vi "对称性.vi"(9 "索引":i32, 10 "定点":dbl, 11 "XY图":cluster{dbl[], dbl[]}[](graph)) -> (3 "对称性":dbl)   [LabVIEW 2020]
uses:
  <vilib>/Analysis/NI_AAL_Geometry.lvlib
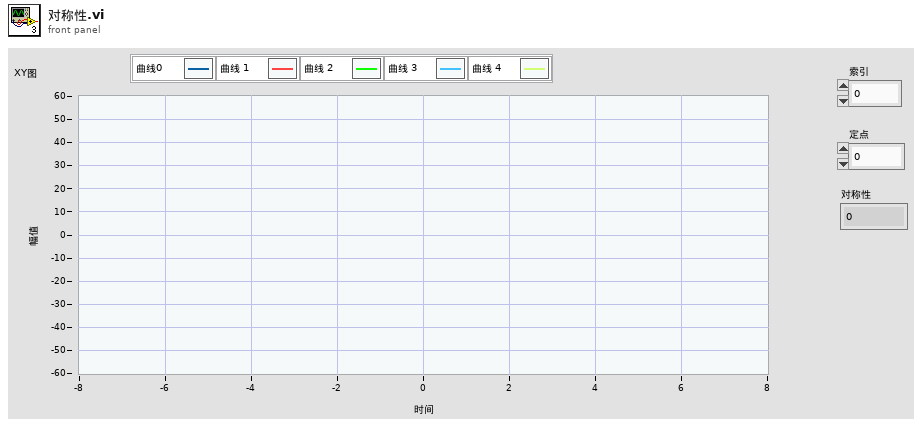
[diagram p1: front panel]
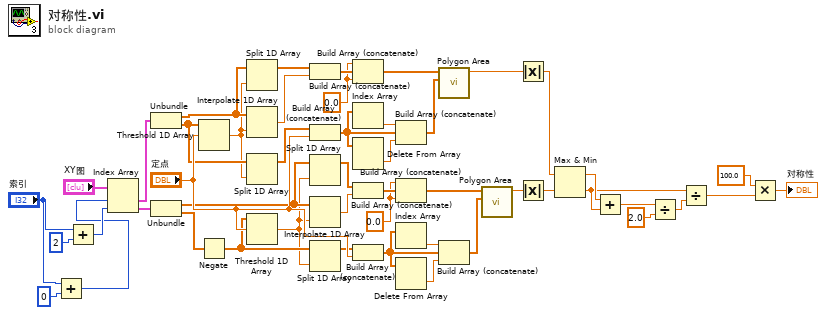
[diagram p0: block diagram]
diagram:
  w31 = 0.0
  w30 = 0.0
  n1 = Add(x="索引", y=0) -> (x+y=w2:i32)
  n2 = Add(x="索引", y=2) -> (x+y=w19:i32)
  n3 = Index Array(array="XY图", index #1=w2, index #2=w19) -> (element #1=w35:cluster{dbl[], dbl[]}, element #2=w21:cluster{dbl[], dbl[]})
  n4 = Unbundle(w35) -> (w32:dbl[], w34:dbl[])
  n5 = Unbundle(w21) -> (w13:dbl[], w33:dbl[])
  n6 = Threshold 1D Array(2:"定点", 3:w34) -> (0:w7:dbl)  [unwired: 1 in]
  n7 = Negate(x=w33) -> (-x=w12:dbl[])
  n8 = Split 1D Array(array=w32, index=w7) -> (first subarray=w11:dbl[])  [unwired: 1 out]
  n9 = Interpolate 1D Array(1:w7, 2:w32) -> (0:w6:dbl)
  n10 = Split 1D Array(array=w34, index=w7) -> (first subarray=w10:dbl[])  [unwired: 1 out]
  n11 = Threshold 1D Array(2:"定点", 3:w12) -> (0:w5:dbl)  [unwired: 1 in]
  n12 = Build Array (concatenate)(w11, w6) -> (w38:dbl[])
  n13 = Build Array (concatenate)(w10, "定点") -> (w40:dbl[])
  n14 = Split 1D Array(array=w13, index=w5) -> (first subarray=w8:dbl[])  [unwired: 1 out]
  n15 = Interpolate 1D Array(1:w5, 2:w13) -> (0:w4:dbl)
  n16 = Split 1D Array(array=w12, index=w5) -> (first subarray=w9:dbl[])  [unwired: 1 out]
  n17 = Build Array (concatenate)(w30, w38, w30) -> (w17:dbl[])
  n18 = Index Array(array=w40) -> (element=w39:dbl)  [unwired: 1 in]
  n19 = Delete From Array(array=w40) -> (deleted portion=w41:dbl)  [unwired: 2 in, 1 out]
  n20 = Build Array (concatenate)(w8, w4) -> (w45:dbl[])
  n21 = Build Array (concatenate)(w9, "定点") -> (w44:dbl[])
  n22 = Build Array (concatenate)(w39, w40, w41) -> (w16:dbl[])
  n23 = Build Array (concatenate)(w31, w45, w31) -> (w15:dbl[])
  n24 = Index Array(array=w44) -> (element=w43:dbl)  [unwired: 1 in]
  n25 = Delete From Array(array=w44) -> (deleted portion=w42:dbl)  [unwired: 2 in, 1 out]
  n26 = call <vilib>:"Polygon Area.vi"("Y"=w16, "X"=w17) -> ("signed area"=w37:dbl)  [unwired: 8 in, 1 out]
  n27 = Build Array (concatenate)(w43, w44, w42) -> (w14:dbl[])
  n28 = call <vilib>:"Polygon Area.vi"("Y"=w14, "X"=w15) -> ("signed area"=w36:dbl)  [unwired: 8 in, 1 out]
  n29 = Absolute Value(x=w37) -> (abs(x)=w29:dbl)
  n30 = Absolute Value(x=w36) -> (abs(x)=w28:dbl)
  n31 = Max & Min(x=w29, y=w28) -> (max(x,y)=w27:dbl, min(x,y)=w24:dbl)
  n32 = Add(x=w27, y=w24) -> (x+y=w26:dbl)
  n33 = Divide(x=w26, y=2.0) -> (x/y=w23:dbl)
  n34 = Divide(x=w24, y=w23) -> (x/y=w22:dbl)
  n35 = Multiply(x=100.0, y=w22) -> (x*y=→"对称性":dbl)
